vi "My Check Polygon Input.vi"(10 "Y In":i32[](array[numeric]), 11 "X In":i32[](array[numeric])) -> (0 "error":i32, 2 "Y Out":i32[](array[numeric]), 3 "X Out":i32[](array[numeric]))   [LabVIEW 2021]
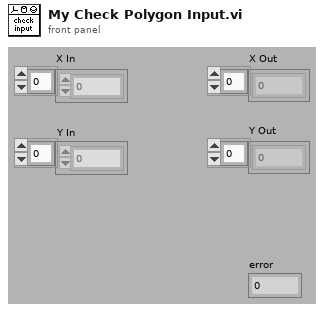
[diagram p1: front panel]
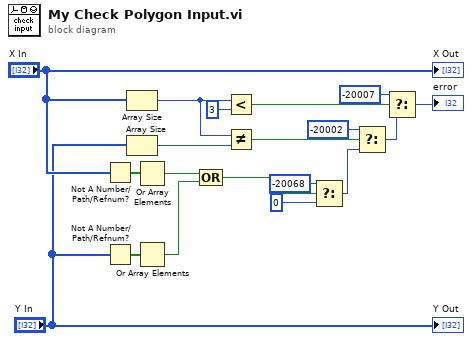
[diagram p0: block diagram]
diagram:
  n1 = Not A Number/Path/Refnum?(number/path/refnum="X In") -> (NaN/Path/Refnum?=w11:bool[])
  n2 = Not A Number/Path/Refnum?(number/path/refnum="Y In") -> (NaN/Path/Refnum?=w10:bool[])
  n3 = Array Size(array="X In") -> (size(s)=w17:i32)
  n4 = Array Size(array="Y In") -> (size(s)=w19:i32)
  n5 = Or Array Elements(Boolean array=w11) -> (logical OR=w9:bool)
  n6 = Or Array Elements(Boolean array=w10) -> (logical OR=w1:bool)
  n7 = Compound Arithmetic op=OR(w9, w1) -> (w6:bool)
  n8 = Less?(x=w17, y=3) -> (x < y?=w5:bool)
  n9 = Not Equal?(x=w17, y=w19) -> (x != y?=w13:bool)
  n10 = Select(t=-20068, s=w6, f=0) -> (s? t:f=w12:i32)
  n11 = Select(t=-20002, s=w13, f=w12) -> (s? t:f=w18:i32)
  n12 = Select(t=-20007, s=w5, f=w18) -> (s? t:f=→"error":i32)
  "X Out" <- "X In"
  "Y Out" <- "Y In"
